vi "test3-MacroWithSubAndPostMessages.vi"(8 "error in":errorcluster, 11 "TestCase in":refnum<class "testcase-CSMResponse.lvclass">) -> (0 "error out":errorcluster, 3 "TestCase out":refnum<class "testcase-CSMResponse.lvclass">)   [LabVIEW 2017, in "testcase-CSMResponse.lvclass"]
uses:
  testcase-CSMResponse.lvclass
  0c6454a9-3719-4e31-9ff6-45b39d38beb6.vi
  2437fcdf-222d-44ea-9250-34e015767128.vi
  src/user.lib/_NEVSTOP/Communicable State Machine(CSM)/AdvanceAPI/CSM - Get Module Attribute.vi
  <vilib>/addons/_JKI Toolkits/VI Tester/TestCase.llb/TestCase.lvclass
  src/user.lib/_NEVSTOP/Communicable State Machine(CSM)/Communicable State Machine.lvlib
  C:/Program Files (x86)/National Instruments/LabVIEW 2017/vi.lib/addons/_JKI Toolkits/VI Tester/TestCase.llb/TestCase.lvclass
panel:
  out "Loopcount":i32
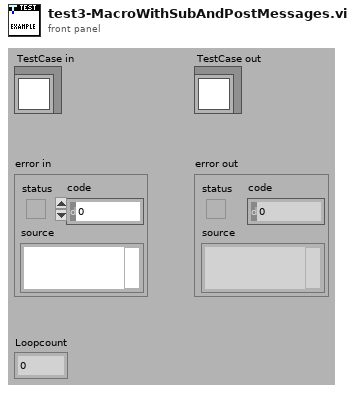
[diagram p1: front panel]
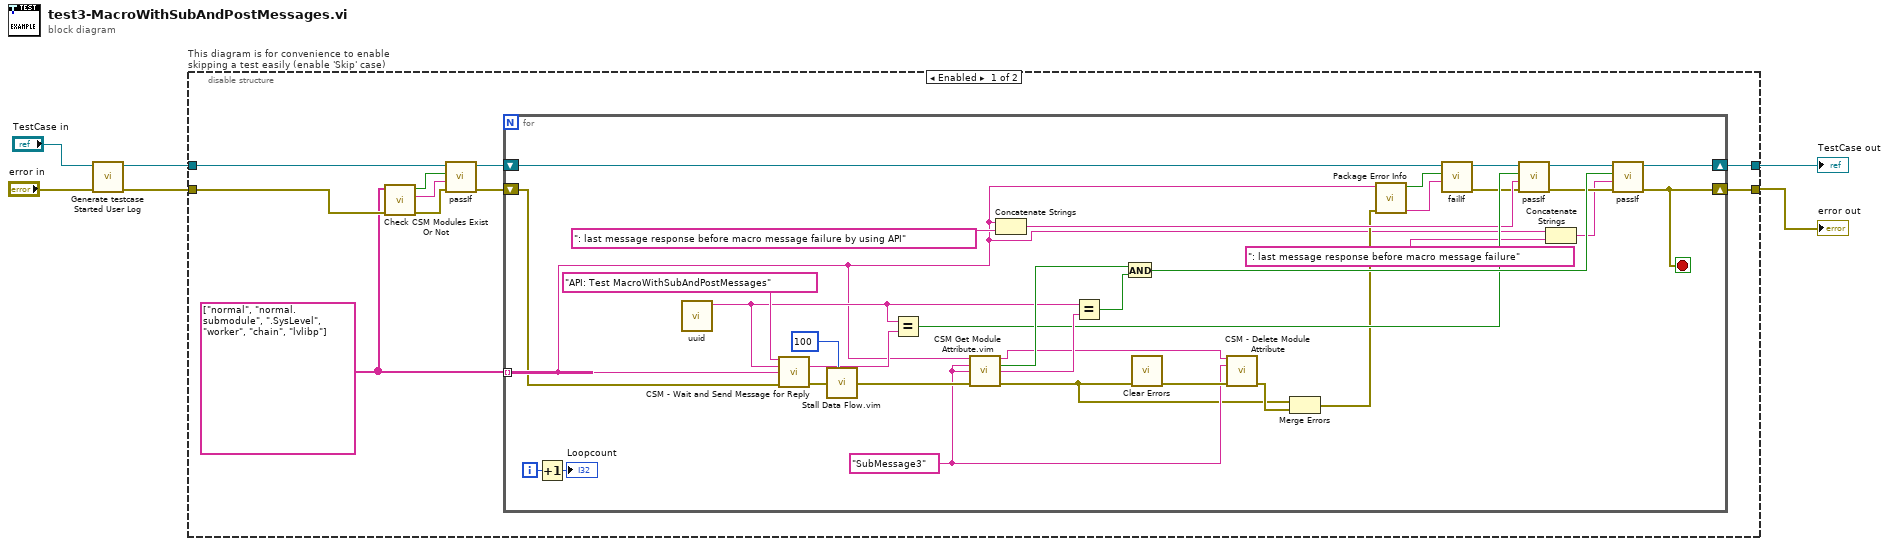
[diagram p0: block diagram]
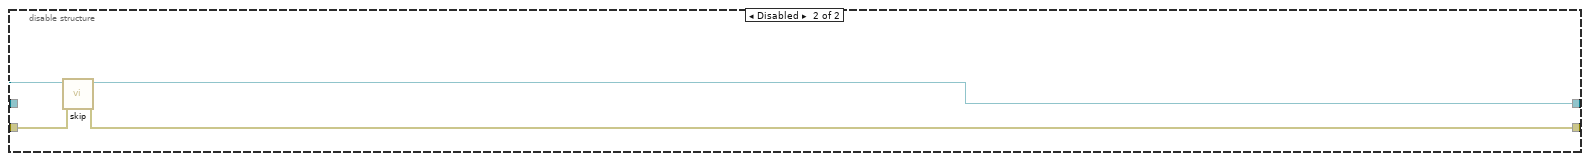
[diagram p2: hidden frame]
diagram:
  n1 = call "Generate testcase Started User Log.vi"("Error In"="error in") -> ("error out"=w1:errorcluster)  [unwired: 10 in]
  n2 = disable-structure "This diagram is for convenience to enable skipping a test easily (enable 'Skip' case)" shown="Enabled" {
    disable-tunnel: "TestCase in" -> [w10 w53]
    disable-tunnel: [w15 w51] -> w2
    disable-tunnel: [w14 w52] -> w4
    disable-tunnel: w1 -> [w7 w50]
    frame Enabled {
      w6 = string[] ["normal", "normal.submodule", ".SysLevel", "worker", "chain", "lvlibp"]
      n3 = call "Check CSM Modules Exist Or Not.vi"("error in"=w7, "CSM names in"=w6) -> ("error out"=w11:errorcluster, "Debug string"=w12:string, "All Modules Exist?"=w13:bool)  [unwired: 7 in]
      n4 = call-dynamic "passIf.vi"("error in (no error)"=w11, "message (\"\")"=w12, "pass"=w13, "TestCase in"=w10) -> ("error out"=w8:errorcluster, "TestCase out"=w9:refnum<class "testcase-CSMResponse.lvclass">)  [unwired: 6 in]
      n5 = for {
        tunnel: w6 -> [w16] mode=indexing
        shift-right: [w36] -> w15
        shift-left: w9 -> [w20]
        shift-right: [w35] -> w14
        shift-left: w8 -> [w29]
        i -> [w49]
        stop <- w35 stop-if-true
        w37 = "SubMessage3" ("Attribute")
        n6 = Increment(x=w49) -> (x+1=→"Loopcount":i32)
        n7 = call "uuid.vi"() -> ("UUID"=w33:string)  [unwired: 11 in]
        n8 = call "CSM - Wait and Send Message for Reply.vi"("State"="API: Test MacroWithSubAndPostMessages", "Arguments (\"\")"=w33, "Target Module"=w16, "Error In (No Error)"=w29) -> ("Response"=w34:string, "error out"=w47:errorcluster)  [unwired: 8 in, 2 out]
        n9 = call "Stall Data Flow.vim"("value in"=w47, "milliseconds to wait"=u32 100) -> ("value out"=w45:errorcluster)  [unwired: 1 out]
        n10 = Equal?(x=w33, y=w34) -> (x = y?=w32:bool)
        n11 = call "CSM Get Module Attribute.vim"("CSM Name"=w16, "Attribute"=w37, "Default Value (Empty Variant)"=w37, "Error In"=w45) -> ("CSM Name (Dup)"=w38:string, "Found"=w44:bool, "Value"=w43:string, "error out"=w27:errorcluster)  [unwired: 7 in, 1 out]
        n12 = Concatenate Strings(w16, ": last message response before macro message failure by using API" ("string")) -> (w25:string)
        n13 = Equal?(x=w33, y=w43) -> (x = y?=w41:bool)
        n14 = And(x=w44, y=w41) -> (x .and. y?=w40:bool)
        n15 = call <vilib>:"Clear Errors.vi"("error in (no error)"=w27) -> ("error out"=w39:errorcluster)  [unwired: 5 in, 1 out]
        n16 = call "CSM - Delete Module Attribute.vi"("CSM Name"=w38, "Attribute"=w37, "Error In"=w39) -> ("error out"=w28:errorcluster)  [unwired: 9 in, 3 out]
        n17 = Merge Errors(w27, w28) -> (w17:errorcluster)
        n18 = call "Package Error Info.vi"("error in"=w17, "String in"=w16) -> ("packed error info out"=w21:string, "error status"=w22:bool)  [unwired: 8 in]
        n19 = call-dynamic "failIf.vi"("message (\"\")"=w21, "fail"=w22, "TestCase in"=w20) -> ("error out"=w18:errorcluster, "TestCase out"=w19:refnum<class "testcase-CSMResponse.lvclass">)  [unwired: 7 in]
        n20 = call-dynamic "passIf.vi"("error in (no error)"=w18, "message (\"\")"=w25, "pass"=w32, "TestCase in"=w19) -> ("error out"=w30:errorcluster, "TestCase out"=w31:refnum<class "testcase-CSMResponse.lvclass">)  [unwired: 6 in]
        n21 = Concatenate Strings(w16, ": last message response before macro message failure" ("string")) -> (w23:string)
        n22 = call-dynamic "passIf.vi"("error in (no error)"=w30, "message (\"\")"=w23, "pass"=w40, "TestCase in"=w31) -> ("error out"=w35:errorcluster, "TestCase out"=w36:refnum<class "testcase-CSMResponse.lvclass">)  [unwired: 6 in]
      }
    }
    frame Disabled {
      # "skip test result while test is under development"
      n23 = call <vilib>:"skip.vi"("error in (no error)"=w50, "TestCase in"=w53) -> ("error out"=w52:errorcluster, "TestCase out"=w51:refnum<class "testcase-CSMResponse.lvclass">)  [unwired: 8 in]
    }
  }
  "error out" <- w4
  "TestCase out" <- w2
